vi "macro_SwerveModPosNew4.vi"   [LabVIEW 2019, in "Trajectory_Library.lvlib"]
uses:
  Rotation2d_CreateAngle.vi
  Translation2d_Create.vi
  Trajectory_Library.lvlib
types:
  T1 = typedef "Trajectory_Library.lvlib/ROTATION2D.ctl" = cluster{"VALUE":dbl, "COS":dbl, "SIN":dbl}
  T2 = typedef "Trajectory_Library.lvlib/SWERVE_DRIVE_MODULE_POSITION.ctl" = cluster{"Distance":dbl, "Angle":T1, "P":bool}
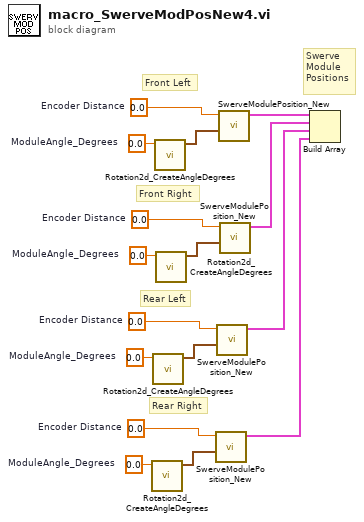
[diagram p0: block diagram]
diagram:
  w4 = 0.0  # ModuleAngle_Degrees
  w6 = 0.0  # Encoder Distance
  w7 = 0.0  # ModuleAngle_Degrees
  w9 = 0.0  # Encoder Distance
  w10 = 0.0  # ModuleAngle_Degrees
  w12 = 0.0  # Encoder Distance
  w14 = 0.0  # ModuleAngle_Degrees
  w16 = 0.0  # Encoder Distance
  # "Front Left"
  # "Swerve\nModule\nPositions"
  # "Rear Right"
  # "Rear Left"
  # "Front Right"
  n1 = call "Rotation2d_CreateAngleDegrees.vi"("Angle_Degrees"=w4) -> ("ROTATION"=w5:T1)  [unwired: 10 in]
  n2 = call "Rotation2d_CreateAngleDegrees.vi"("Angle_Degrees"=w7) -> ("ROTATION"=w8:T1)  [unwired: 10 in]
  n3 = call "Rotation2d_CreateAngleDegrees.vi"("Angle_Degrees"=w14) -> ("ROTATION"=w15:T1)  [unwired: 10 in]
  n4 = call "Rotation2d_CreateAngleDegrees.vi"("Angle_Degrees"=w10) -> ("ROTATION"=w11:T1)  [unwired: 10 in]
  n5 = call "SwerveModulePosition_New.vi"("ROTATION"=w5, "Distance"=w6) -> ("SWERVE_DRIVE_MODULE_POSITION"=w1:T2)  [unwired: 9 in]
  n6 = call "SwerveModulePosition_New.vi"("ROTATION"=w8, "Distance"=w9) -> ("SWERVE_DRIVE_MODULE_POSITION"=w2:T2)  [unwired: 9 in]
  n7 = call "SwerveModulePosition_New.vi"("ROTATION"=w15, "Distance"=w16) -> ("SWERVE_DRIVE_MODULE_POSITION"=w13:T2)  [unwired: 9 in]
  n8 = call "SwerveModulePosition_New.vi"("ROTATION"=w11, "Distance"=w12) -> ("SWERVE_DRIVE_MODULE_POSITION"=w3:T2)  [unwired: 9 in]
  n9 = Build Array(w13, w3, w2, w1) -> ()  [unwired: 1 out]
